vi "Destroy.vi"(8 "error in (no error)":errorcluster, 11 "ClientBase in":refnum<class "ClientBase.lvclass">) -> (0 "error out":errorcluster)   [LabVIEW 2020, in "ClientBaseLib.lvlib" / "ClientBase.lvclass"]
uses:
  ClientBase.lvclass
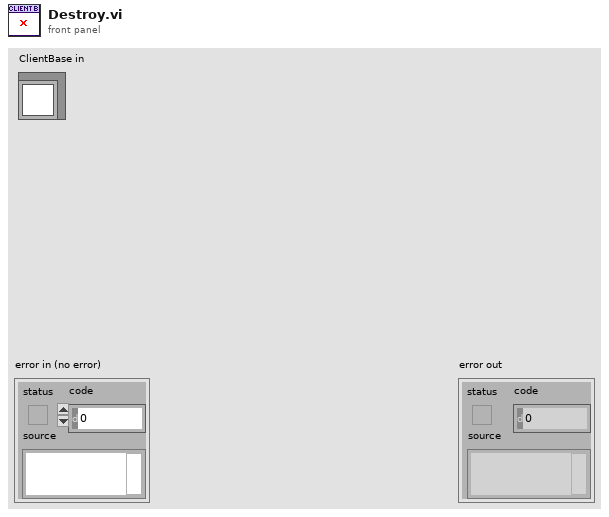
[diagram p1: front panel]
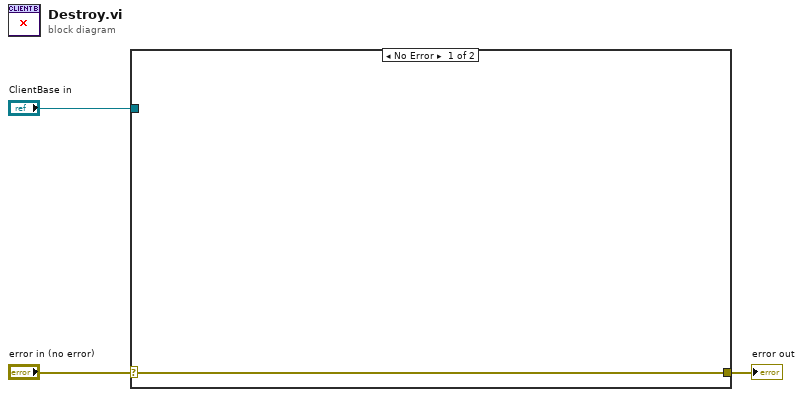
[diagram p0: block diagram]
diagram:
  n1 = case shown="No Error" "error in (no error)" {
    selector: "error in (no error)" -> [w4 w5]
    tunnel: [w4 w5] -> w2
    tunnel: "ClientBase in" -> [_ _]
    frame No Error {
    }
    frame Error {
    }
  }
  "error out" <- w2
